vi "vipm_unInstallPackagesbyName.vi"(8 "error in (no error)":errorcluster, 11 "CommandLine":string[](array[string])) -> (0 "error out":errorcluster, 2 "test details":string, 3 "output to action":string)   [LabVIEW 2014]
uses:
  <userlib>/_OpenG.lib/array/array.llb/Index 1D Array Elements (String)__ogtk.vi
  <vilib>/JKI/VIPM API/VIPM API_vipm_api.lvlib
  _lvcicd/_lvcicd_support_2014.lvlib
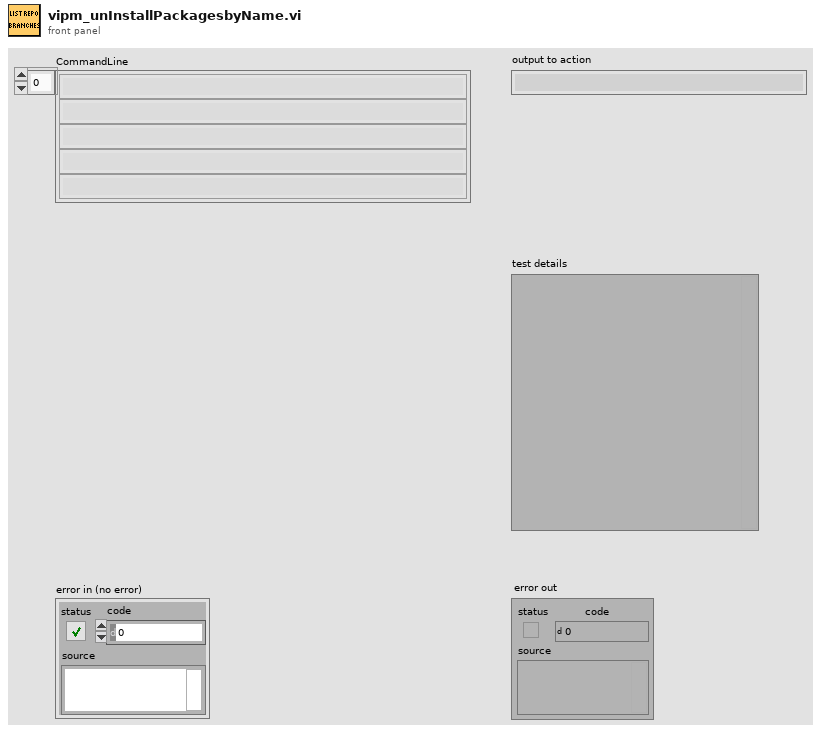
[diagram p1: front panel]
types:
  T1 = typedef "VIPM API_vipm_api.lvlib/Library Contents Cluster_vipm_api.ctl" = cluster{"Package Name":string, "Version":string, "Display Name":string, "Repository Name":string, "Company Name":string, "License Type":string, "Installed":bool, "Deprecated":bool, "Dependency or Conflict Problem":bool, "Downloaded":bool}
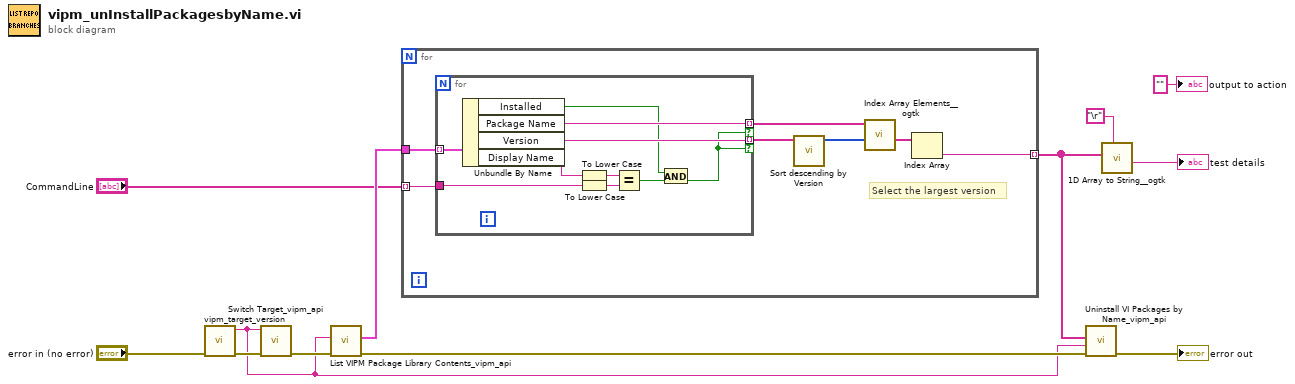
[diagram p0: block diagram]
diagram:
  n1 = call "vipm_target_version.vi"() -> ("vipm Taget version"=w2:string)  [unwired: 11 in]
  n2 = call <vilib>:"Switch Target_vipm_api.vi"("error in (no error)"="error in (no error)", "LabVIEW Version"=w2) -> ("error out"=w3:errorcluster)  [unwired: 9 in]
  n3 = call <vilib>:"List VIPM Package Library Contents_vipm_api.vi"("error in (no error)"=w3, "LabVIEW Version"=w2) -> ("error out"=w8:errorcluster, "Library Contents []"=w7:T1[])  [unwired: 7 in, 1 out]
  n4 = for {
    tunnel: w7 -> [w18]
    tunnel: "CommandLine" -> [w17] mode=indexing
    tunnel: [w12] -> w5 mode=indexing
    # "Select the largest version"
    n5 = for {
      tunnel: w18 -> [w28] mode=indexing
      tunnel: w17 -> [w26]
      tunnel: [w25] -> w16 mode=indexing if=w20
      tunnel: [w24] -> w15 mode=indexing if=w20
      n6 = Unbundle By Name(w28) -> ("Installed"=w19:bool, "Package Name"=w24:string, "Version"=w25:string, "Display Name"=w27:string)
      n7 = To Lower Case(string=w27) -> (all lower case string=w22:string)
      n8 = To Lower Case(string=w26) -> (all lower case string=w21:string)
      n9 = Equal?(x=w22, y=w21) -> (x = y?=w23:bool)
      n10 = And(x=w19, y=w23) -> (x .and. y?=w20:bool)
    }
    n11 = call "Sort descending by Version.vi"("Array"=w16) -> ("Sorted Pointers"=w14:i32[])  [unwired: 10 in]
    n12 = call-poly <userlib>:"Index Array Elements__ogtk.vi"("indices"=w14, "array"=w15) -> ("elements"=w13:string[])  [unwired: 9 in]
    n13 = Index Array(array=w13) -> (element=w12:string)  [unwired: 1 in]
  }
  n14 = call <vilib>:"Uninstall VI Packages by Name_vipm_api.vi"("error in (no error)"=w8, "LabVIEW Version"=w2, "Package Names to Uninstall []"=w5) -> ("error out"=→"error out":errorcluster)  [unwired: 8 in]
  n15 = call <userlib>:"1D Array to String__ogtk.vi"("delimiter (Tab)"="\r", "Array of Strings"=w5) -> ("delimited string"=→"test details":string)  [unwired: 9 in]
  "output to action" <- "" ("output to action")
